vi "Module Loop.vi"(8 "error in (no error)":errorcluster, 11 "DAQmxAI in":refnum<class "DAQmxAI.lvclass">) -> (0 "error out":errorcluster, 3 "DAQmxAI out":refnum<class "DAQmxAI.lvclass">)   [LabVIEW 2023, in "VolatusDAQ.lvlib" / "DAQmxAI.lvclass"]
uses:
  DAQmxAI.lvclass
  DAQmxAI.lvclass/DAQmxAI.ctl
  Volatus/Module/Module.lvclass
  Volatus/MessageQ/MessageQ.lvclass
  <resource>/objmgr/daqmx.rc
  lv-vecto/Vecto/Group DBL/Group DBL.lvclass
  C:/dev/volatus/mts-volatus-super/libs/lv-volatus/Volatus/Module/Module.lvclass
  C:/dev/volatus/mts-volatus-super/libs/lv-volatus/VolatusDAQ/DAQmxAI/DAQmxAI.lvclass
  C:/dev/volatus/mts-volatus-super/libs/lv-vecto/Vecto/Group/Group.lvclass
  C:/dev/volatus/mts-volatus-super/libs/lv-vecto/Vecto/Group DBL/Group DBL.lvclass
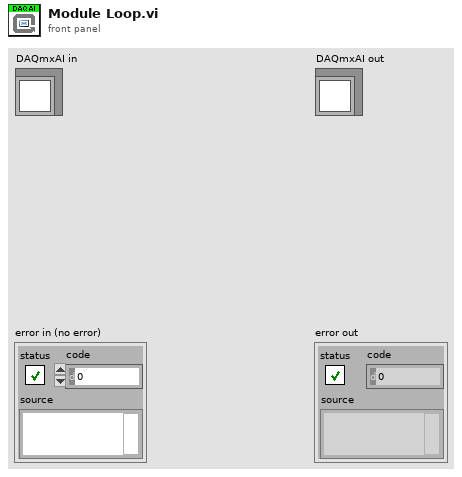
[diagram p1: front panel]
types:
  T1 = enum32{"Invalid", "Standard", "Closed", "Hidden", "Minimized", "Maximized"}
  T2 = typedef "CmdDigitalMultiple.lvlib/Data.ctl" = cluster{"values":T3[]}
  T3 = typedef "CmdDigital.lvlib/Data.ctl" = cluster{"channel":string, "value":bool}
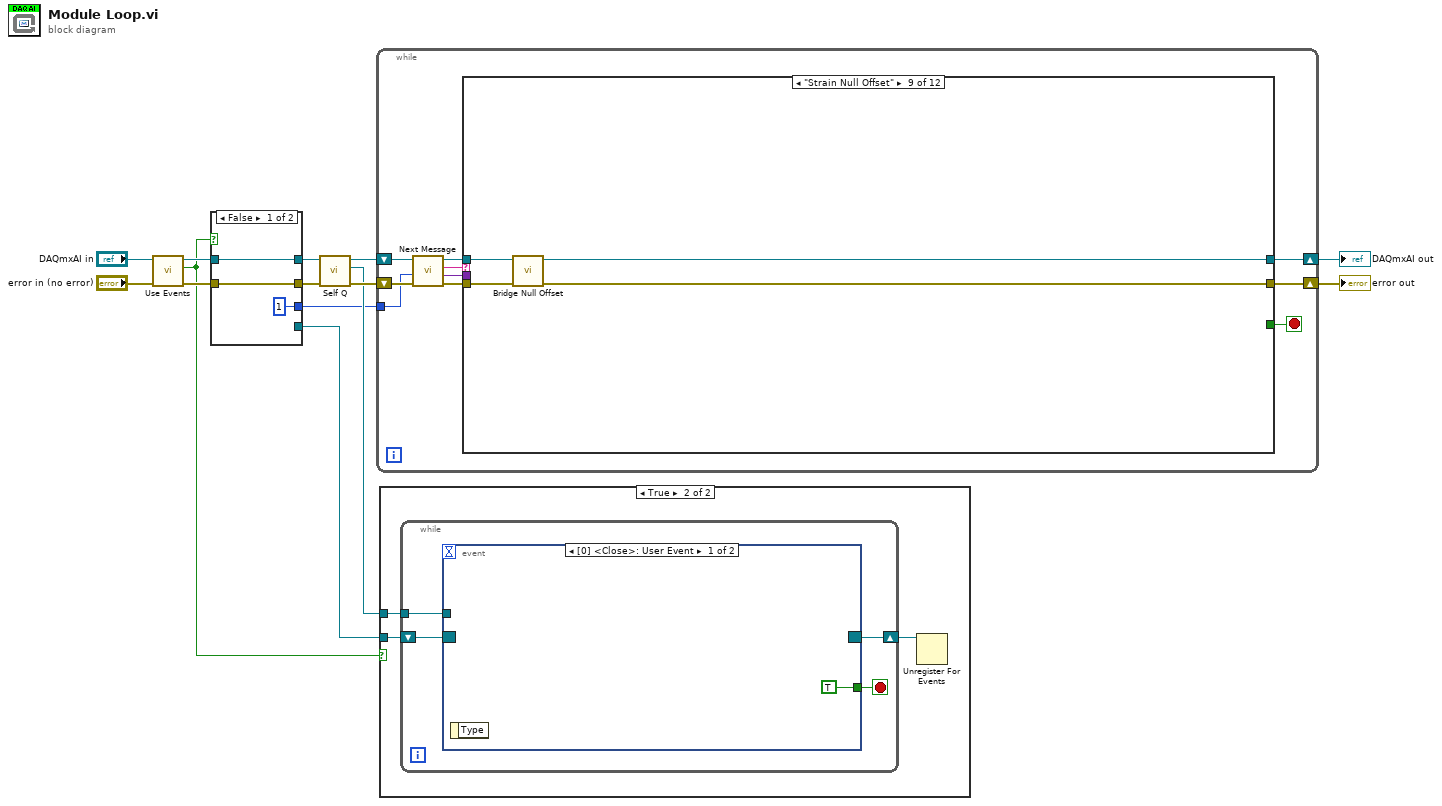
[diagram p0: block diagram]
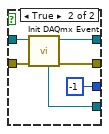
[diagram p2: hidden frame]
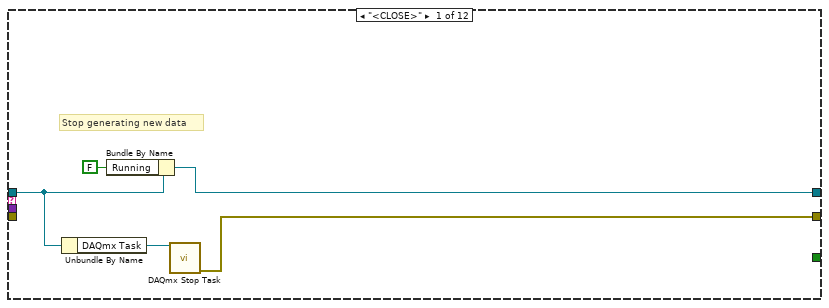
[diagram p3: hidden frame]
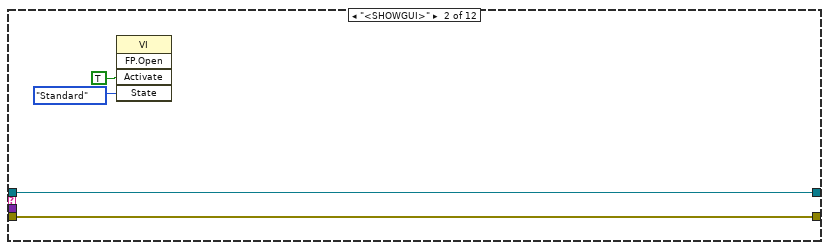
[diagram p4: hidden frame]
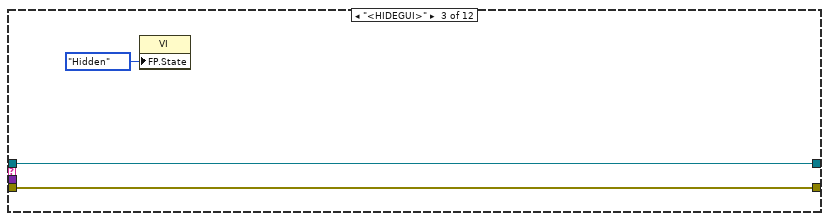
[diagram p5: hidden frame]
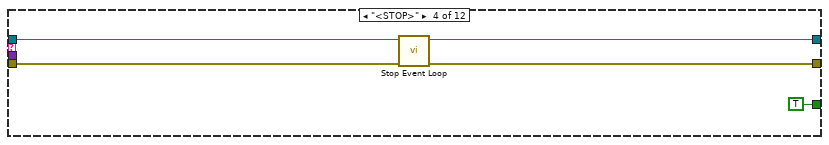
[diagram p6: hidden frame]
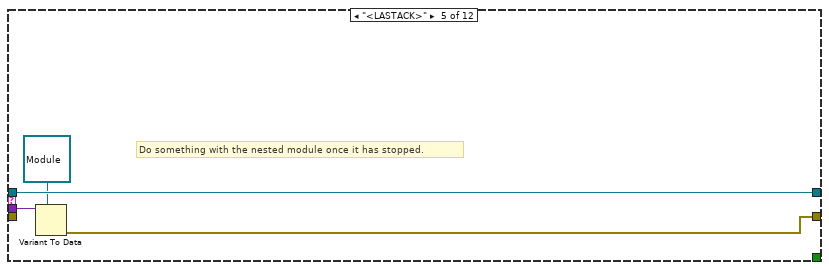
[diagram p7: hidden frame]
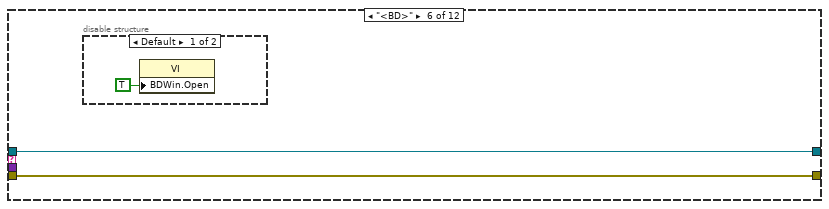
[diagram p8: hidden frame]
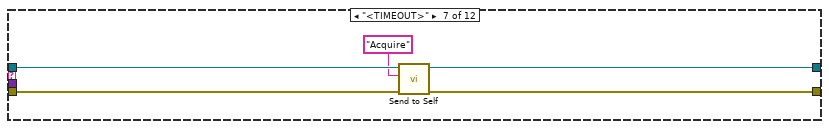
[diagram p10: hidden frame]
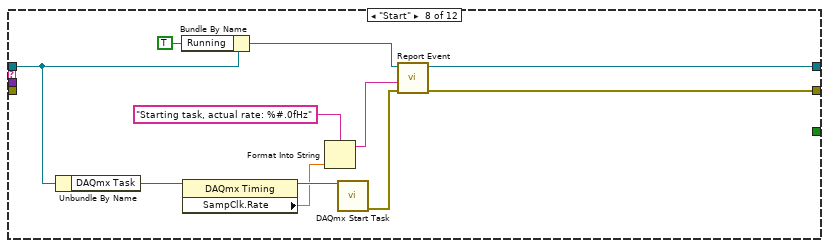
[diagram p11: hidden frame]
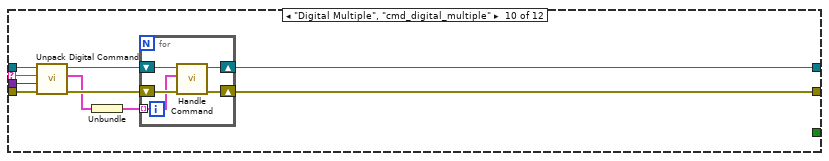
[diagram p12: hidden frame]
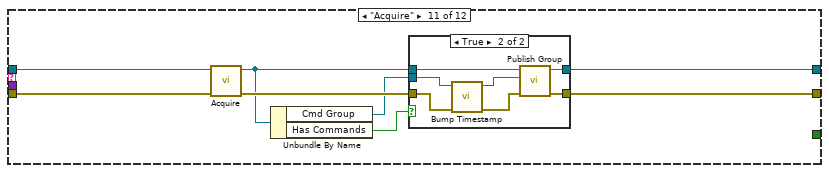
[diagram p13: hidden frame]
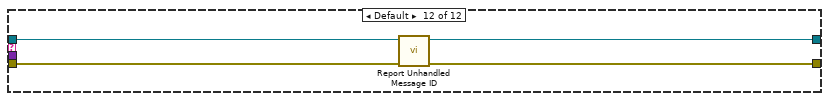
[diagram p15: hidden frame]
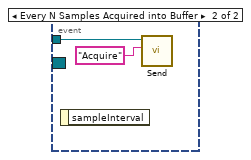
[diagram p17: hidden frame]
diagram:
  n1 = call "Use Events.vi"("error in (no error)"="error in (no error)", "DAQmxAI in"="DAQmxAI in") -> ("error out"=w5:errorcluster, "Use Events"=w2:bool, "DAQmxAI out"=w3:refnum<class "DAQmxAI.lvclass">)  [unwired: 7 in]
  n2 = case shown="False" w2 {
    tunnel: [w15 w22] -> w10
    tunnel: [w16 w21] -> w9
    tunnel: [_ w20] -> w8
    tunnel: w5 -> [w15 w19]
    tunnel: w3 -> [w16 w18]
    tunnel: [1 -1] -> w1
    frame False {
    }
    frame True {
      n3 = call "Init DAQmx Event.vi"("error in (no error)"=w19, "DAQmxAI in"=w18) -> ("error out"=w22:errorcluster, "DAQmxAI out"=w21:refnum<class "DAQmxAI.lvclass">, "Event Reg"=w20:refnum<event-registration>)  [unwired: 7 in]
    }
  }
  n4 = call "Self Q.vi"("Module in"=w9) -> ("Self Q"=w6:refnum<class "MessageQ.lvclass">, "Module out"=w7:refnum<class "DAQmxAI.lvclass">)  [unwired: 9 in]
  n5 = while {
    shift-right: [w27] -> w12
    shift-left: w7 -> [w32]
    shift-right: [w26] -> w11
    shift-left: w10 -> [w31]
    tunnel: w1 -> [w23]
    stop <- w25 stop-if-true
    n6 = call "Next Message.vi"("error in (no error)"=w31, "Timeout/Period ms (-1)"=w23, "Module in"=w32) -> ("error out"=w30:errorcluster, "Data"=w24:variant, "ID"=w29:string, "Module out"=w28:refnum<class "DAQmxAI.lvclass">)  [unwired: 5 in]
    n7 = case shown="\"Strain Null Offset\"" w29 {
      selector: w29 -> [_ _ _ _ _ _ _ _ _ w80 _ _]
      tunnel: w30 -> [_ w40 w43 w49 _ w54 w61 _ w75 w82 w98 w112]
      tunnel: w28 -> [w35 w41 w44 w46 w53 w55 w59 w72 w76 w83 w97 w110]
      tunnel: [w37 w41 w44 w45 w53 w55 w58 w63 w73 w85 w95 w109] -> w27
      tunnel: [w33 w40 w43 w47 w50 w54 w60 w65 w74 w84 w92 w111] -> w26
      tunnel: [_ _ _ TRUE _ _ _ _ _ _ _ _] -> w25
      tunnel: w24 -> [_ _ _ _ w52 _ _ _ _ w81 _ _]
      frame "<CLOSE>" {
        # "Stop generating new data"
        n8 = Unbundle By Name(w35) -> ("DAQmx Task"=w34:refnum<k21>)
        n9 = Bundle By Name(cluster=w35, "Running"=FALSE) -> (w37:refnum<class "DAQmxAI.lvclass">)
        n10 = call <vilib>:"DAQmx Stop Task.vi"("task/channels in"=w34) -> ("error out"=w33:errorcluster)  [unwired: 13 in, 1 out]
      }
      frame "<SHOWGUI>" {
        n11 = invoke class="VI" method="FP.Open"("Activate"=TRUE ("Activate?"), "State"=T1."Standard") -> ()  [unwired: 3 in, 5 out]
      }
      frame "<HIDEGUI>" {
        n12 = property class="VI"("FP.State"=T1."Hidden" ("Front Panel Window:State")) -> ()  [unwired: 2 in, 2 out]
      }
      frame "<STOP>" {
        n13 = call "Stop Event Loop.vi"("error in (no error)"=w49, "DAQmxAI in"=w46) -> ("error out"=w47:errorcluster, "DAQmxAI out"=w45:refnum<class "DAQmxAI.lvclass">)  [unwired: 8 in]
      }
      frame "<LASTACK>" {
        # "Do something with the nested module once it has stopped."
        n14 = Variant To Data(type=refnum<class "Module.lvclass"> refnum ("Volatus:Module"), Variant=w52) -> (error out=w50:errorcluster)  [unwired: 1 in, 1 out]
      }
      frame "<BD>" {
        n15 = disable-structure shown="Default" {
          frame condition #0 (active) {
            n16 = property class="VI"("BDWin.Open"=TRUE ("Block Diagram Window:Open")) -> ()  [unwired: 2 in, 2 out]
          }
          frame condition #1 {
          }
        }
      }
      frame "<TIMEOUT>" {
        n17 = call "Send to Self.vi"("error in (no error)"=w61, "Message ID"="Acquire", "Module in"=w59) -> ("error out"=w60:errorcluster, "Module out"=w58:refnum<class "DAQmxAI.lvclass">)  [unwired: 7 in]
      }
      frame "Start" {
        n18 = Unbundle By Name(w72) -> ("DAQmx Task"=w69:refnum<k21>)
        n19 = Bundle By Name(cluster=w72, "Running"=TRUE) -> (w64:refnum<class "DAQmxAI.lvclass">)
        n20 = property class="DAQmx Timing"(reference=w69) -> (reference out=w68:refnum<k21>, "SampClk.Rate"=w66:dbl)  [unwired: 1 in, 1 out]
        n21 = Format Into String(format string="Starting task, actual rate: %#.0fHz", w66) -> (resulting string=w62:string)  [unwired: 2 in, 1 out]
        n22 = call <vilib>:"DAQmx Start Task.vi"("task/channels in"=w68) -> ("error out"=w71:errorcluster)  [unwired: 13 in, 1 out]
        n23 = call "Report Event.vi"("error in (no error)"=w71, "Message"=w62, "Module in"=w64) -> ("error out"=w65:errorcluster, "Module out"=w63:refnum<class "DAQmxAI.lvclass">)  [unwired: 7 in]
      }
      frame "Strain Null Offset" {
        n24 = call "Bridge Null Offset.vi"("error in (no error)"=w75, "DAQmxAI in"=w76) -> ("error out"=w74:errorcluster, "DAQmxAI out"=w73:refnum<class "DAQmxAI.lvclass">)  [unwired: 8 in]
      }
      frame "Digital Multiple", "cmd_digital_multiple" {
        n25 = call "Unpack Digital Command.vi"("error in (no error)"=w82, "Data"=w81, "Type"=w80, "Module in"=w83) -> ("error out"=w79:errorcluster, "CmdDigitalMultiple"=w77:T2, "Module out"=w78:refnum<class "DAQmxAI.lvclass">)  [unwired: 3 in, 2 out]
        n26 = Unbundle(w77) -> ("values"=w86:T3[])
        n27 = for {
          tunnel: w86 -> [w87] mode=indexing
          shift-right: [w88] -> w85
          shift-left: w78 -> [w91]
          shift-right: [w89] -> w84
          shift-left: w79 -> [w90]
          n28 = call "Handle Command.vi"("error in (no error)"=w90, "Data"=w87, "DAQmxAI in"=w91) -> ("error out"=w89:errorcluster, "DAQmxAI out"=w88:refnum<class "DAQmxAI.lvclass">)  [unwired: 7 in]
        }
      }
      frame "Acquire" {
        n29 = call "Acquire.vi"("error in (no error)"=w98, "DAQmxAI in"=w97) -> ("error out"=w99:errorcluster, "DAQmxAI out"=w96:refnum<class "DAQmxAI.lvclass">)  [unwired: 8 in]
        n30 = Unbundle By Name(w96) -> ("Cmd Group"=w94:refnum<class "Group DBL.lvclass">, "Has Commands"=w93:bool)
        n31 = case shown="True" w93 {
          tunnel: w99 -> [w100 w103]
          tunnel: w96 -> [w101 w108]
          tunnel: [w101 w107] -> w95
          tunnel: w94 -> [_ w105]
          tunnel: [w100 w106] -> w92
          frame False {
          }
          frame True {
            n32 = call "Bump Timestamp.vi"("error in (no error)"=w103, "Group in"=w105) -> ("error out"=w102:errorcluster, "Group out"=w104:refnum<class "Group DBL.lvclass">)  [unwired: 8 in]
            n33 = call "Publish Group.vi"("error in (no error)"=w102, "Group"=w104, "Module in"=w108) -> ("error out"=w106:errorcluster, "Module out"=w107:refnum<class "DAQmxAI.lvclass">)  [unwired: 7 in]
          }
        }
      }
      frame Default {
        n34 = call "Report Unhandled Message ID.vi"("error in (no error)"=w112, "Module in"=w110) -> ("error out"=w111:errorcluster, "Module out"=w109:refnum<class "DAQmxAI.lvclass">)  [unwired: 8 in]
      }
    }
  }
  "error out" <- w11
  "DAQmxAI out" <- w12
  n35 = case shown="True" w2 {
    tunnel: w8 -> [_ w115]
    tunnel: w6 -> [_ w114]
    frame False {
    }
    frame True {
      n36 = while {
        tunnel: w114 -> [w118]
        shift-right: [w117] -> w113
        shift-left: w115 -> [w119]
        stop <- w116 stop-if-true
        n37 = event shown="[0] <Close>: User Event" {
          selector: w119 -> [_ _]
          dyn-events: [_ _] -> w117
          timeout: _ -> [_ _]
          tunnel: w118 -> [_ w122]
          tunnel: [TRUE _] -> w116
          event User Event {
            n38 = event-data() -> ()  [unwired: 1 in, 1 out]
          }
          event Every N Samples Acquired into Buffer {
            n39 = event-data() -> ()  [unwired: 1 in, 1 out]
            n40 = call "Send.vi"("ID"="Acquire", "MessageQ in"=w122) -> ()  [unwired: 8 in, 2 out]
          }
        }
      }
      n41 = Unregister For Events(event registration refnum=w113) -> ()  [unwired: 1 in, 1 out]
    }
  }
